vi "Connect Path.vi"(8 "error in":errorcluster, 11 "2525 in":refnum<class "2525.lvclass">) -> (0 "error out":errorcluster, 3 "2525 out":refnum<class "2525.lvclass">)   [LabVIEW 2019, in "2525.lvlib" / "2525.lvclass"]
uses:
  Library/2525.lvclass
  Library/2525.lvclass/2525.ctl
  <instrlib>/niSwitch/niSwitch.llb/niSwitch Connect Channels (Single).vi
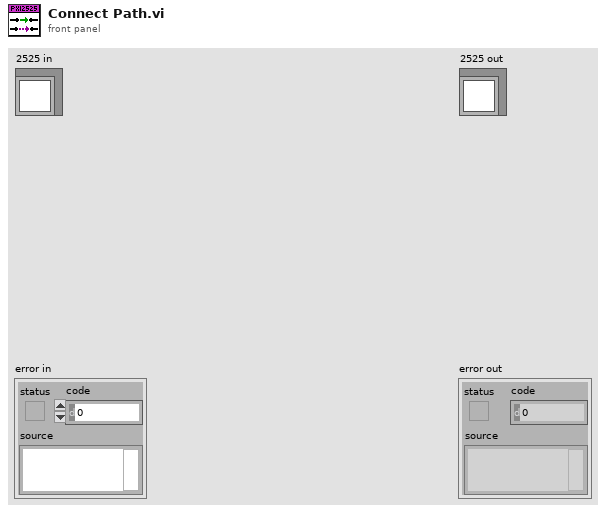
[diagram p1: front panel]
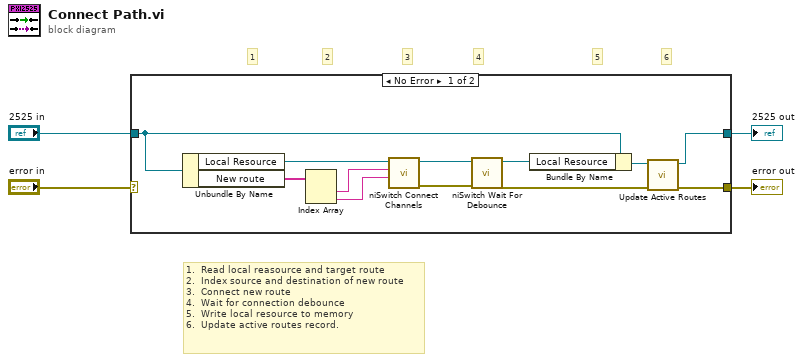
[diagram p0: block diagram]
diagram:
  # "1.  Read local reasource and target route\n2.  Index source and destination of new route\n3.  Connect new route\n4.  Wait for connection debounce\n5.  Write local resource to memory\n6.  Update active routes record."
  # "6"
  # "5"
  # "4"
  # "3"
  # "2"
  # "1"
  n1 = case shown="No Error" "error in" {
    selector: "error in" -> [_ w18]
    tunnel: [w6 w18] -> w3
    tunnel: [w5 w17] -> w1
    tunnel: "2525 in" -> [w12 w17]
    frame No Error {
      n2 = Unbundle By Name(w12) -> ("Local Resource"=w16:refnum<k15>, "New route"=w15:string[])
      n3 = Index Array(array=w15) -> (element #1=w14:string, element #2=w13:string)  [unwired: 2 in]
      n4 = call-poly <instrlib>:"niSwitch Connect Channels.vi"("channel 2"=w13, "channel 1"=w14, "instrument handle"=w16) -> ("error out"=w11:errorcluster, "instrument handle out"=w10:refnum<k15>)  [unwired: 7 in]
      n5 = call <instrlib>:"niSwitch Wait For Debounce.vi"("error in (no error)"=w11, "instrument handle"=w10) -> ("error out"=w7:errorcluster, "instrument handle out"=w9:refnum<k15>)  [unwired: 8 in]
      n6 = Bundle By Name(cluster=w12, "Local Resource"=w9) -> (w8:refnum<class "2525.lvclass">)
      n7 = call "Update Active Routes.vi"("error in"=w7, "2525 in"=w8) -> ("error out"=w6:errorcluster, "2525 out"=w5:refnum<class "2525.lvclass">)  [unwired: 8 in]
    }
    frame Error {
    }
  }
  "error out" <- w3
  "2525 out" <- w1
